vi "CALC_MATH_FUNC.vi"(0 "VISA IN":refnum<visa-resource-name>, 5 "error in":errorcluster, 7 "Channel":i32, 11 "Combo Box":string(combo)="NORM") -> (14 "VISA Out":refnum<visa-resource-name>, 19 "error out":errorcluster)   [LabVIEW 2018, in "PNA-X.lvlib"]
doc: "CALCulate<cnum>:MATH:FUNCtion <char> \n(Read-Write) Sets math operations on the currently selected measurement and the trace stored in \nmemory. (There MUST be a trace stored in Memory. See CALC:MATH MEM) \nSee Critical Note \nParameters \n<cnum> Channel number of the measurement. There must be a selected measurement \non that channel. If unspecified, <cnum> is set to 1. \n<char> The math operation to be applied. Choose from the following: \nNORMal Trace data only \nADD Data + Memory \nSUBTract Data - Memory \nMULTiply Data * Memory \nDIVide Data / Memory \n1544\n\nExamples CALC:MATH:FUNC NORM \ncalculate2:math:function subtract \nQuery Syntax CALCulate<cnum>:MATH:FUNCtion? \nReturn Type Character \nDefault NORMal"
uses:
  PNA-X.lvlib
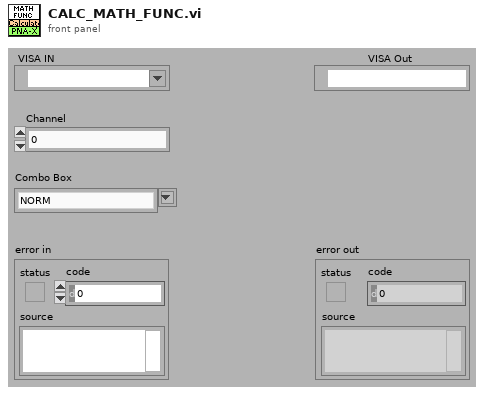
[diagram p1: front panel]
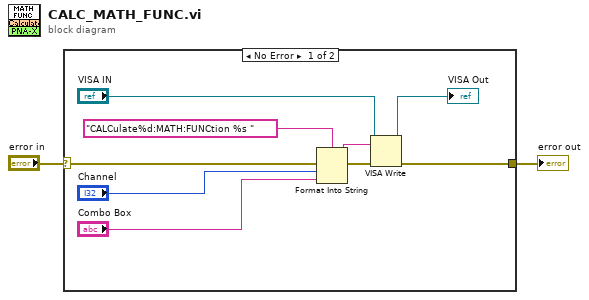
[diagram p0: block diagram]
diagram:
  n1 = case shown="No Error" "error in" {
    selector: "error in" -> [w11 w12]
    tunnel: [w6 w12] -> w1
    frame No Error {
      n2 = Format Into String(format string="CALCulate%d:MATH:FUNCtion %s " ("Cmdline"), error in=w11, "Channel", "Combo Box") -> (resulting string=w9:string, error out=w10:errorcluster)  [unwired: 1 in]
      n3 = VISA Write(VISA resource name="VISA IN", write buffer=w9, error in (no error)=w10) -> (VISA resource name out=→"VISA Out":refnum<visa-resource-name>, error out=w6:errorcluster)  [unwired: 1 out]
    }
    frame Error {
    }
  }
  "error out" <- w1
